vi "mean calc.vi"(11 "Cluster in":T1) -> (3 "Cluster out":T1)   [LabVIEW 2021]
uses:
  b0ee5c3b-add9-40aa-821e-fc9f63331328.vi
  <vilib>/Analysis/baseanly.llb/Mean (DBL).vi
  <vilib>/Array/Sort 2D Array - Pop Stack.vi
  <vilib>/Array/Sort 2D Array - Push Stack.vi
  b0ee5c3b-add9-40aa-821e-fc9f63331328.vi/269d4b3b-47f5-49e3-8884-44851e4dd9d5.vi
  b0ee5c3b-add9-40aa-821e-fc9f63331328.vi/6d99389c-673d-4efb-bf33-19b32bcf4cf8.vi
  <vilib>/Analysis/NI_AALBase.lvlib
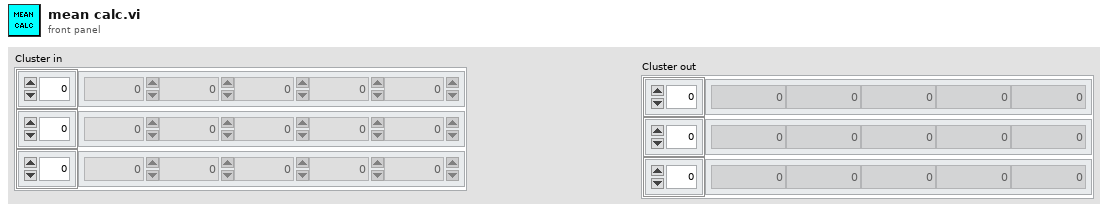
[diagram p1: front panel]
types:
  T1 = cluster{"Array":dbl[], "Array":dbl[], "Array":dbl[]}
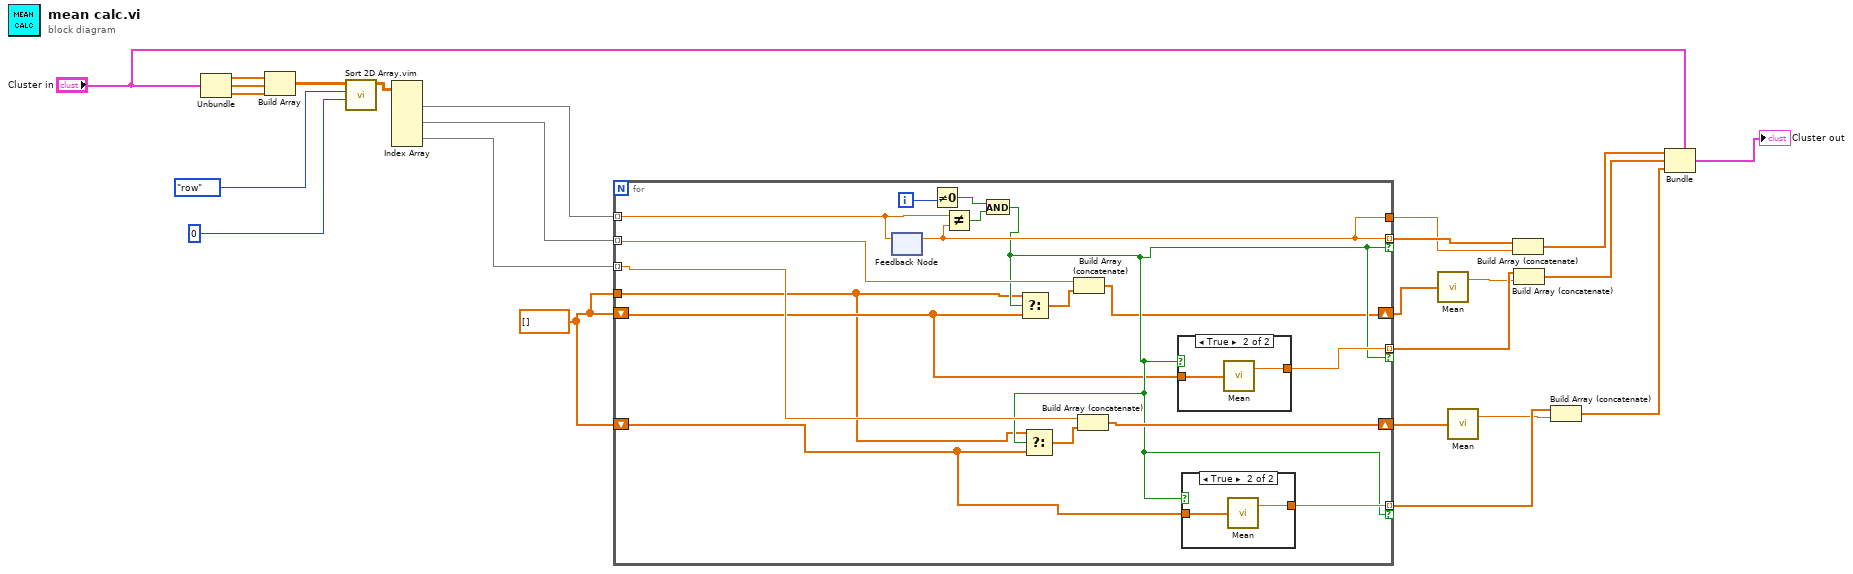
[diagram p0: block diagram]
diagram:
  w1 = dbl[] [] ("t")
  n1 = Unbundle("Cluster in") -> ("Array"=w24:dbl[], "Array"=w23:dbl[], "Array"=w22:dbl[])
  n2 = Build Array(w24, w23, w22) -> (w21:dbl[][])
  n3 = call "Sort 2D Array.vim"("index"=0, "dimension to index (column)"=enum16{"column", "row"}."row", "2D array"=w21) -> ("sorted 2D array"=w17:dbl[][])  [unwired: 7 in, 1 out]
  n4 = Index Array(array=w17) -> (element #1=w15:dbl[], element #2=w14:dbl[], element #3=w13:dbl[])  [unwired: 6 in]
  n5 = for {
    tunnel: w15 -> [w41] mode=indexing
    tunnel: w14 -> [w40] mode=indexing
    tunnel: w13 -> [w36] mode=indexing
    tunnel: [w38] -> w9 mode=indexing if=w29
    tunnel: [w33] -> w7 mode=indexing if=w29
    tunnel: [w35] -> w11 mode=indexing if=w29
    tunnel: [w33] -> w6
    shift-right: [w28] -> w2
    shift-left: w1 -> [w27]
    tunnel: w1 -> [w25]
    shift-right: [w34] -> w12
    shift-left: w1 -> [w26]
    i -> [w32]
    n6 = feedback #1() -> (w33:dbl)  [unwired: 1 in]
    n7 = feedback-in #1(w41) -> ()
    n8 = Not Equal To 0?(x=w32) -> (x != 0?=w31:bool)
    n9 = Not Equal?(x=w41, y=w33) -> (x != y?=w30:bool)
    n10 = And(x=w31, y=w30) -> (x .and. y?=w29:bool)
    n11 = Select(t=w25, s=w29, f=w27) -> (s? t:f=w39:dbl[])
    n12 = Select(t=w25, s=w29, f=w26) -> (s? t:f=w37:dbl[])
    n13 = Build Array (concatenate)(w40, w39) -> (w28:dbl[])
    n14 = Build Array (concatenate)(w36, w37) -> (w34:dbl[])
    n15 = case shown="True" w29 {
      tunnel: w27 -> [_ w45]
      tunnel: [_ w44] -> w38
      frame False {
      }
      frame True {
        n16 = call-poly <vilib>:"Mean.vi"("X"=w45) -> ("mean"=w44:dbl)  [unwired: 1 out]
      }
    }
    n17 = case shown="True" w29 {
      tunnel: w26 -> [_ w43]
      tunnel: [_ w42] -> w35
      frame False {
      }
      frame True {
        n18 = call-poly <vilib>:"Mean.vi"("X"=w43) -> ("mean"=w42:dbl)  [unwired: 1 out]
      }
    }
  }
  n19 = call-poly <vilib>:"Mean.vi"("X"=w2) -> ("mean"=w8:dbl)  [unwired: 1 out]
  n20 = call-poly <vilib>:"Mean.vi"("X"=w12) -> ("mean"=w10:dbl)  [unwired: 1 out]
  n21 = Build Array (concatenate)(w7, w6) -> (w5:dbl[])
  n22 = Build Array (concatenate)(w9, w8) -> (w4:dbl[])
  n23 = Build Array (concatenate)(w11, w10) -> (w3:dbl[])
  n24 = Bundle(cluster="Cluster in", "Array"=w5, "Array"=w4, "Array"=w3) -> (→"Cluster out":T1)
